vi "setFPGA.vi"(10 "FPGA":refnum<class "FPGA.lvclass">, 11 "ModbusSubnetDTxDataFIFO in":refnum<class "ModbusSubnetDTxDataFIFO.lvclass">) -> (3 "ModbusSubnetDTxDataFIFO out":refnum<class "ModbusSubnetDTxDataFIFO.lvclass">)   [LabVIEW 2016, in "ModbusSubnetDTxDataFIFO.lvclass"]
uses:
  ModbusSubnetDTxDataFIFO.lvclass
  FPGA/FPGA.lvclass
  ModbusSubnetDTxDataFIFO.lvclass/ModbusSubnetDTxDataFIFO.ctl
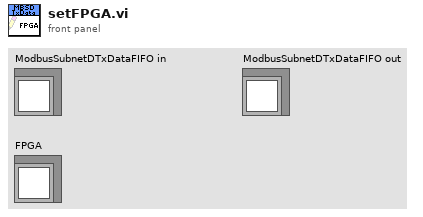
[diagram p1: front panel]
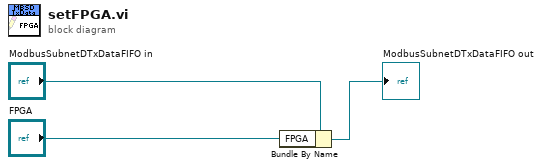
[diagram p0: block diagram]
diagram:
  n1 = Bundle By Name(cluster="ModbusSubnetDTxDataFIFO in", "FPGA"="FPGA") -> (→"ModbusSubnetDTxDataFIFO out":refnum<class "ModbusSubnetDTxDataFIFO.lvclass">)
